vi "Image-characteristics.vi"(8 "error in":errorcluster, 10 "Buffer element in":T1 {"Temperature characteristics"."Stand. dev. temperature" format="%#.1f"; "Temperature characteristics"."Min. temperature" format="%#.0f"; "Temperature characteristics"."Max. temperature" format="%#.0f"; "Temperature characteristics"."Average temperature" format="%#.0f"}, 11 "Analysis params. ref. in":refnum<data-value>) -> (0 "error IO":errorcluster, 2 "Buffer element":T1 {"Temperature characteristics"."Stand. dev. temperature" format="%#.1f"; "Temperature characteristics"."Min. temperature" format="%#.0f"; "Temperature characteristics"."Max. temperature" format="%#.0f"; "Temperature characteristics"."Average temperature" format="%#.0f"}, 3 "Analysis params. ref.":refnum<data-value>)   [LabVIEW 2013, in "CameraVision.lvlib" / "CV-Main.lvclass"]
uses:
  CV-Main.lvclass
  Analysis/CV-Analysis.lvclass
  Buffers/Storage-buffer.ctl
  <vilib>/vision/Image Controls.llb/IMAQ Image.ctl
  Temperature/Temperature-characteristics.ctl
  Analysis/Characteristics-cluster.ctl
  Analysis/CV-Analysis.lvclass/CV-Analysis.ctl
  Analysis/Read Image characteristics.vi
  <vilib>/vision/NI_Vision_Development_Module.lvlib
  Temperature/CV-Temperature.lvclass
  Buffers/CV-Buffers.lvclass
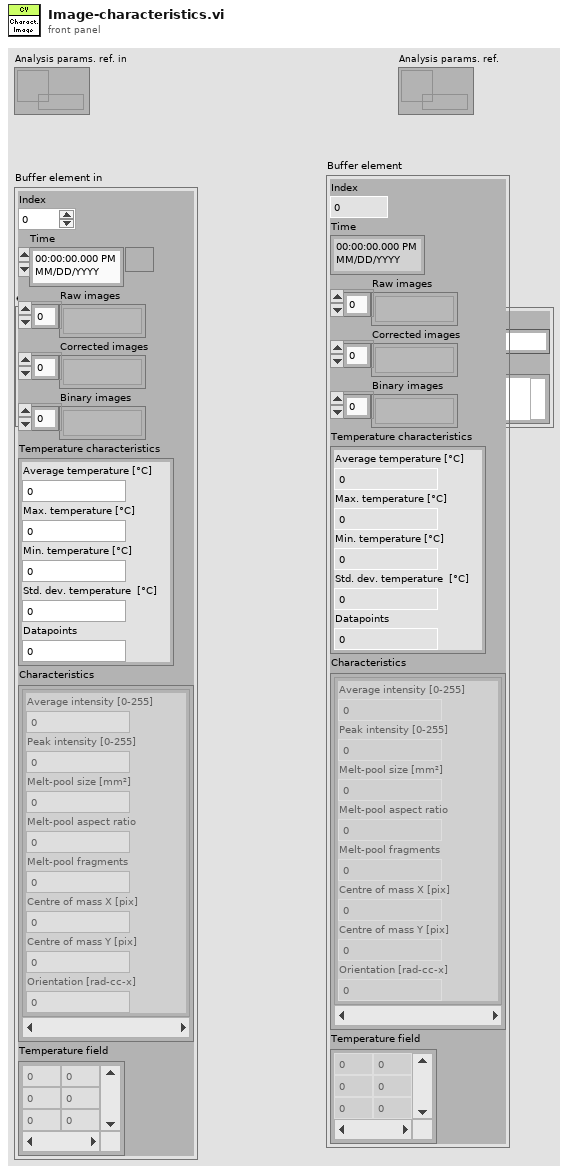
[diagram p1: front panel]
types:
  T1 = typedef "CameraVision.lvlib/CV-Buffers.lvclass/Storage-buffer.ctl" = cluster{"Index":i32, "Time":timestamp, "Raw images":T2[], "Corrected images":T2[], "Binary images":T2[], "Temperature characteristics":T3, "Characteristics":T4[], "Temperature field":dbl[][]}
  T2 = typedef "IMAQ Image.ctl" = refnum<image>
  T3 = typedef "CameraVision.lvlib/CV-Temperature.lvclass/Temperature-characteristics.ctl" = cluster{"Average temperature ":dbl, "Max. temperature":dbl, "Min. temperature":dbl, "Stand. dev. temperature":dbl, "Datapoints":dbl}
  T4 = typedef "CameraVision.lvlib/CV-Analysis.lvclass/Characteristics-cluster.ctl" = cluster{"Average intensity":dbl, "Peak intensity":dbl, "Melt-pool size":dbl, "Melt-pool aspect ratio":dbl, "Melt-pool fragments":dbl, "Centre of mass X":dbl, "Centre of mass Y":dbl, "Orientation":dbl}
  T5 = cluster{"Mean Value":sgl, "Standard Variation":sgl, "Minimal Value":sgl, "Maximal Value":sgl, "Area (calibrated)":sgl, "Area (pixels)":u32, "%":sgl, "Calibration Valid":bool}
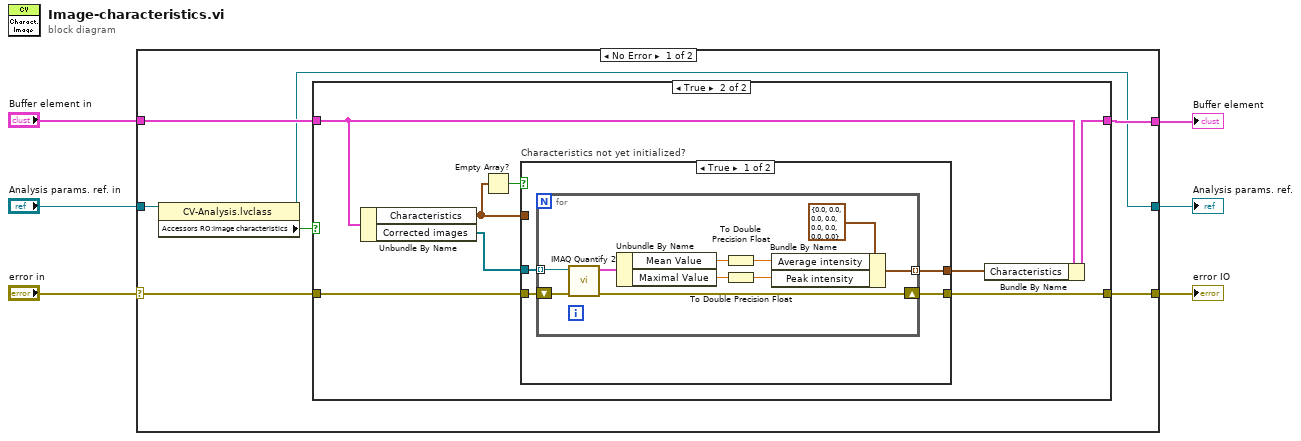
[diagram p0: block diagram]
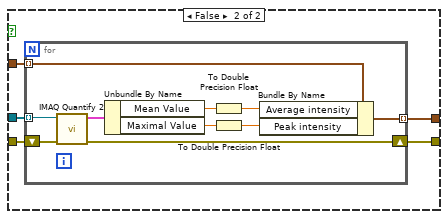
[diagram p3: hidden frame]
diagram:
  n1 = case shown="No Error" "error in" {
    selector: "error in" -> [w9 w55]
    tunnel: [w7 w55] -> w5
    tunnel: "Buffer element in" -> [w13 w53]
    tunnel: "Analysis params. ref. in" -> [w12 w54]
    tunnel: [w8 w54] -> w2
    tunnel: [w10 w53] -> w1
    frame No Error {
      n2 = property class="CV-Analysis.lvclass"(reference=w12) -> (reference out=w8:refnum<data-value>, "Accessors RO:Image characteristics"=w11:bool)  [unwired: 1 in, 1 out]
      n3 = case shown="True" w11 {
        tunnel: w13 -> [w15 w22]
        tunnel: [w14 w23] -> w7
        tunnel: [w15 w17] -> w10
        tunnel: w9 -> [w14 w21]
        frame False {
        }
        frame True {
          n4 = Unbundle By Name(w22) -> ("Characteristics"=w19:T4[], "Corrected images"=w18:T2[])
          n5 = Empty Array?(array=w19) -> (empty?=w20:bool)
          n6 = case "Characteristics not yet initialized?" shown="True" w20 {
            tunnel: w18 -> [w27 w42]
            tunnel: [w26 w41] -> w23
            tunnel: [w25 w40] -> w16
            tunnel: w21 -> [w24 w39]
            tunnel: w19 -> [_ w38]
            frame True {
              n7 = for {
                tunnel: w27 -> [w33] mode=indexing
                tunnel: [w30] -> w25 mode=indexing
                shift-right: [w29] -> w26
                shift-left: w24 -> [w36]
                n8 = call "IMAQ Quantify 2"("error in (no error)"=w36, "Image"=w33) -> ("error out"=w29:errorcluster, "Global Report"=w37:T5)  [unwired: 7 in, 1 out]
                n9 = Unbundle By Name(w37) -> ("Mean Value"=w35:sgl, "Maximal Value"=w34:sgl)
                n10 = To Double Precision Float(number=w35) -> (double precision float=w32:dbl)
                n11 = To Double Precision Float(number=w34) -> (double precision float=w31:dbl)
                n12 = Bundle By Name(cluster=T4 {"Average intensity"=0.0, "Peak intensity"=0.0, "Melt-pool size"=0.0, "Melt-pool aspect ratio"=0.0, "Melt-pool fragments"=0.0, "Centre of mass X"=0.0, "Centre of mass Y"=0.0, "Orientation"=0.0} ("Characteristics"), "Average intensity"=w32, "Peak intensity"=w31) -> (w30:T4)
              }
            }
            frame False {
              n13 = for {
                tunnel: w42 -> [w48] mode=indexing
                tunnel: [w45] -> w40 mode=indexing
                shift-right: [w44] -> w41
                shift-left: w39 -> [w51]
                tunnel: w38 -> [w43] mode=indexing
                n14 = call "IMAQ Quantify 2"("error in (no error)"=w51, "Image"=w48) -> ("error out"=w44:errorcluster, "Global Report"=w52:T5)  [unwired: 7 in, 1 out]
                n15 = Unbundle By Name(w52) -> ("Mean Value"=w50:sgl, "Maximal Value"=w49:sgl)
                n16 = To Double Precision Float(number=w50) -> (double precision float=w47:dbl)
                n17 = To Double Precision Float(number=w49) -> (double precision float=w46:dbl)
                n18 = Bundle By Name(cluster=w43, "Average intensity"=w47, "Peak intensity"=w46) -> (w45:T4)
              }
            }
          }
          n19 = Bundle By Name(cluster=w22, "Characteristics"=w16) -> (w17:T1)
        }
      }
    }
    frame Error {
    }
  }
  "error IO" <- w5
  "Buffer element" <- w1
  "Analysis params. ref." <- w2
